vi "Target Level Conversion.vi"(0 "Target Level[]":dbl[](array[numeric]), 1 "PowerUp?":bool, 2 "Negative Target Level?":bool) -> (4 "Target Level[] OUT":dbl[](array[numeric]))   [LabVIEW 2024, in "devicePowerSequencerCoreLogic.lvlib"]
uses:
  devicePowerSequencerCoreLogic.lvlib
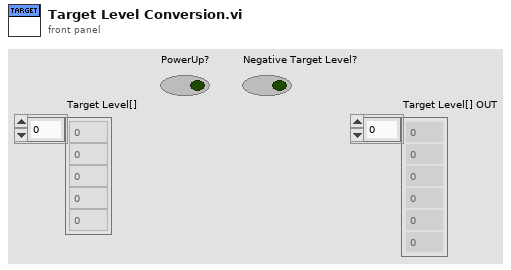
[diagram p1: front panel]
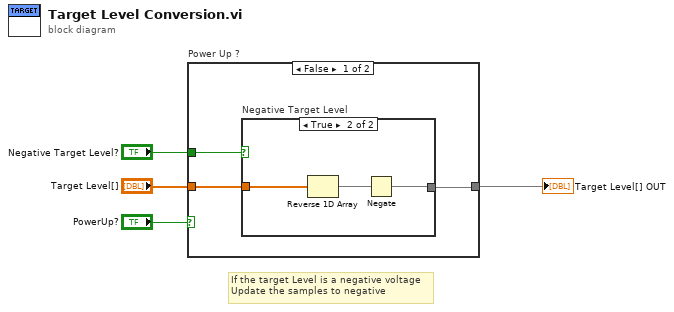
[diagram p0: block diagram]
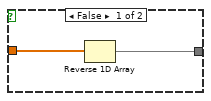
[diagram p2: hidden frame]
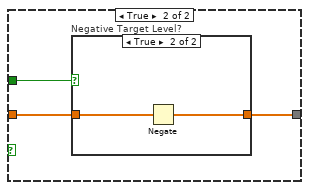
[diagram p3: hidden frame]
diagram:
  # "If the target Level is a negative voltage\nUpdate the samples to negative"
  n1 = case "Power Up ?" shown="False" "PowerUp?" {
    tunnel: "Negative Target Level?" -> [w7 w15]
    tunnel: "Target Level[]" -> [w6 w14]
    tunnel: [w5 w13] -> w2
    frame False {
      n2 = case "Negative Target Level" shown="True" w7 {
        tunnel: w6 -> [w9 w12]
        tunnel: [w8 w10] -> w5
        frame False {
          n3 = Reverse 1D Array(array=w9) -> (reversed array=w8:dbl[])
        }
        frame True {
          n4 = Reverse 1D Array(array=w12) -> (reversed array=w11:dbl[])
          n5 = Negate(x=w11) -> (-x=w10:dbl[])
        }
      }
    }
    frame True {
      n6 = case "Negative Target Level?" shown="True" w15 {
        tunnel: w14 -> [w16 w18]
        tunnel: [w16 w17] -> w13
        frame False {
          # "Pass the samples"
        }
        frame True {
          n7 = Negate(x=w18) -> (-x=w17:dbl[])
        }
      }
    }
  }
  "Target Level[] OUT" <- w2
